vi "GetControlValue_Boolean.vi"(8 "error in (no error)":errorcluster, 9 "Expected Data Type":bool, 10 "Control Label":string, 11 "CtlLookup In":T1) -> (0 "error out":errorcluster, 2 "Value":bool, 3 "CtlLookup Out":T1)   [LabVIEW 2020, in "CtlReferences.lvlib" / "CtlReferences.lvclass"]
doc: "This VI uses the GetControlByReference to get the specified control as a bool"
uses:
  CtlReferences.lvclass
  TypeDefs/CtlLookup.ctl
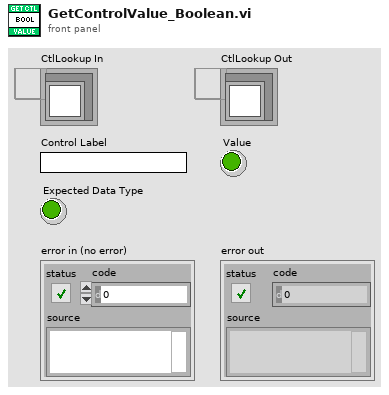
[diagram p1: front panel]
types:
  T1 = typedef "CtlReferences.lvlib/CtlReferences.lvclass/CtlLookup.ctl" = refnum<data-value>
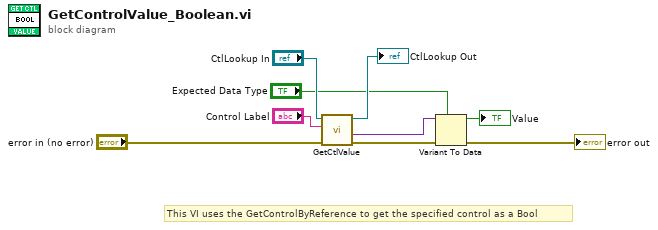
[diagram p0: block diagram]
diagram:
  # "This VI uses the GetControlByReference to get the specified control as a Bool"
  n1 = call "GetCtlValue.vi"("Error in"="error in (no error)", "CtlName In"="Control Label", "CtlLookup In"="CtlLookup In") -> ("error out"=w1:errorcluster, "Value"=w4:variant, "CtlLookup Out"=→"CtlLookup Out":T1)  [unwired: 6 in]
  n2 = Variant To Data(error in=w1, type="Expected Data Type", Variant=w4) -> (data=→"Value":bool, error out=→"error out":errorcluster)
